vi "_PC_Spectrafilter get_roi_data.vi"(6 "SigProc":bool, 8 "error in (no error)":errorcluster, 10 "rule parameter":T1, 11 "file tree ref in":refnum<vi>) -> (0 "error out":errorcluster, 2 "s/n ratio array":dbl[](array[numeric]), 3 "file ref array":path[](array[path]))   [LabVIEW 2018]
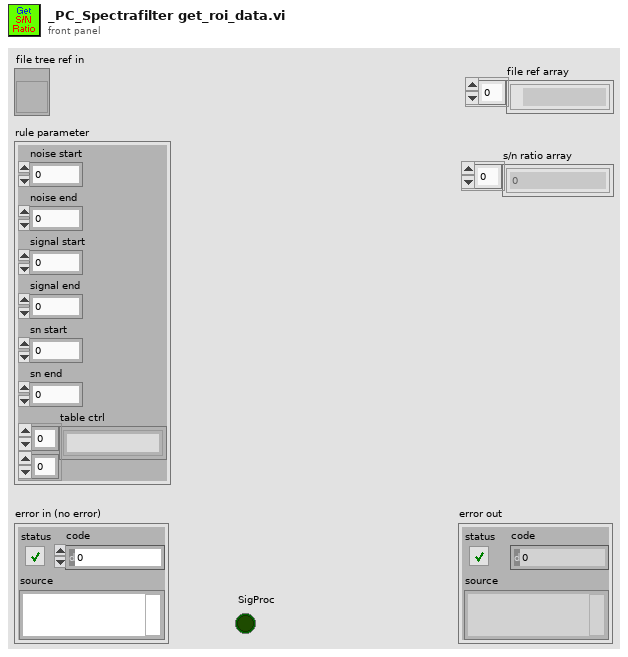
[diagram p1: front panel]
types:
  T1 = cluster{"noise start":dbl, "noise end":dbl, "signal start":dbl, "signal end":dbl, "sn start":dbl, "sn end":dbl, "table ctrl":string[][]}
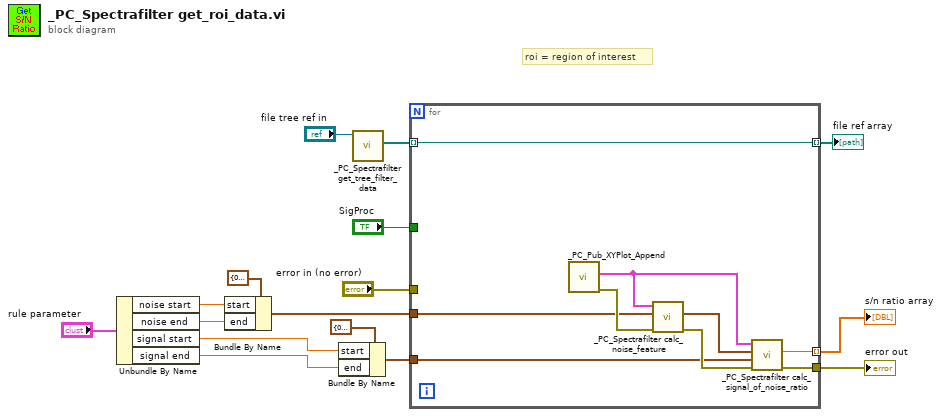
[diagram p0: block diagram]
diagram:
  # "roi = region of interest"
  n1 = Unbundle By Name("rule parameter") -> ("noise start"=w8:dbl, "noise end"=w7:dbl, "signal start"=w6:dbl, "signal end"=w5:dbl)
  n2 = Bundle By Name(cluster=cluster{"start":dbl, "end":dbl} {"start"=0.0, "end"=0.0} ("noise range"), "start"=w8, "end"=w7) -> (w4:cluster{"start":dbl, "end":dbl})
  n3 = Bundle By Name(cluster=cluster{"start":dbl, "end":dbl} {"start"=0.0, "end"=0.0} ("signal range"), "start"=w6, "end"=w5) -> (w3:cluster{"start":dbl, "end":dbl})
  n4 = call "_PC_Spectrafilter get_tree_filter_data.vi"("file tree ref"="file tree ref in") -> ("datas path"=w16:path[])  [unwired: 9 in, 1 out]
  n5 = for {
    tunnel: w16 -> [w17] mode=indexing
    tunnel: "SigProc" -> [_]
    tunnel: "error in (no error)" -> [_]
    tunnel: [w20] -> w2
    tunnel: [w21] -> w12 mode=indexing
    tunnel: w4 -> [w19]
    tunnel: w3 -> [w18]
    tunnel: [w17] -> w1 mode=indexing
    n6 = call "_PC_Pub_XYPlot_Append.vi"() -> ("error out"=w22:errorcluster, "Spectrum out"=w23:cluster{"X":dbl[], "Y":sgl[]})  [unwired: 9 in, 1 out]
    n7 = call "_PC_Spectrafilter calc_noise_feature.vi"("error in (no error)"=w22, "noise range"=w19, "spectrum data"=w23) -> ("error out"=w24:errorcluster, "noise feature"=w25:cluster{"noise diff":sgl, "median":dbl})  [unwired: 7 in]
    n8 = call "_PC_Spectrafilter calc_signal_of_noise_ratio.vi"("error in (no error)"=w24, "signal range"=w18, "noise feature"=w25, "Spectrum in"=w23) -> ("error out"=w20:errorcluster, "ratio"=w21:dbl)  [unwired: 6 in]
  }
  "error out" <- w2
  "s/n ratio array" <- w12
  "file ref array" <- w1
